vi "WriteAllData.vi"(8 "error in (no error)":errorcluster, 10 "Input":string[](array[string]), 11 "Sensor in":refnum<class "Sensor.lvclass">) -> (0 "error out":errorcluster, 3 "Sensor out":refnum<class "Sensor.lvclass">)   [LabVIEW 2014, in "Sensors.lvlib" / "Sensor.lvclass"]
uses:
  Sensor.lvclass
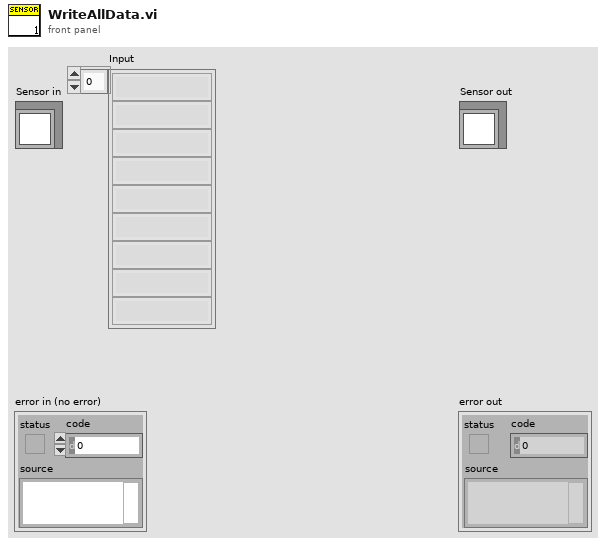
[diagram p1: front panel]
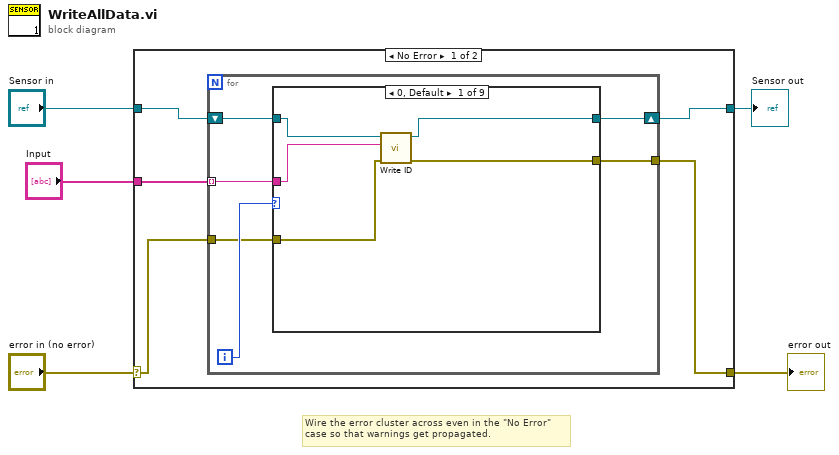
[diagram p0: block diagram]
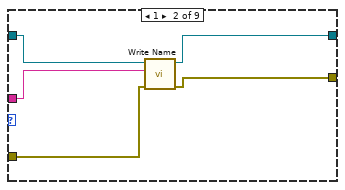
[diagram p2: hidden frame]
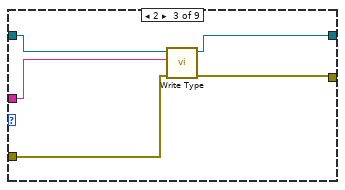
[diagram p3: hidden frame]
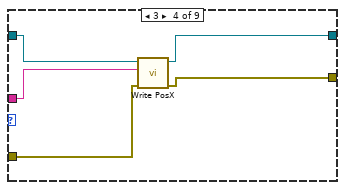
[diagram p4: hidden frame]
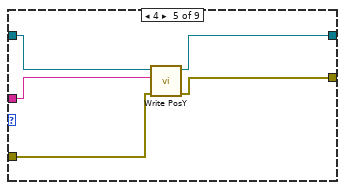
[diagram p5: hidden frame]
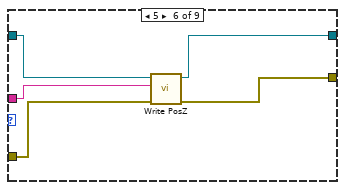
[diagram p6: hidden frame]
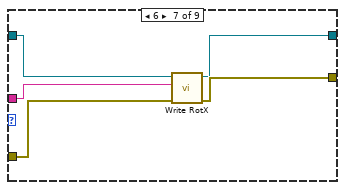
[diagram p7: hidden frame]
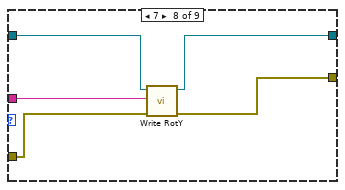
[diagram p8: hidden frame]
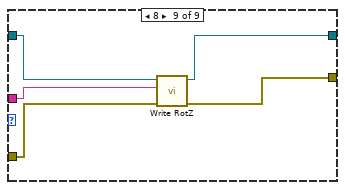
[diagram p9: hidden frame]
diagram:
  # "Wire the error cluster across even in the \"No Error\"\ncase so that warnings get propagated."
  n1 = case shown="No Error" "error in (no error)" {
    selector: "error in (no error)" -> [w7 w63]
    tunnel: [w6 w63] -> w1
    tunnel: [w9 w62] -> w3
    tunnel: "Sensor in" -> [w10 w62]
    tunnel: "Input" -> [w8 _]
    frame No Error {
      n2 = for {
        tunnel: w8 -> [w15] mode=indexing
        tunnel: w7 -> [w12]
        tunnel: [w11] -> w6
        shift-right: [w13] -> w9
        shift-left: w10 -> [w14]
        i -> [w16]
        n3 = case shown="0, Default" w16 {
          tunnel: w15 -> [w19 w24 w29 w35 w40 w45 w50 w53 w59]
          tunnel: w14 -> [w21 w26 w30 w36 w41 w46 w51 w56 w61]
          tunnel: [w20 w25 w31 w33 w38 w43 w47 w55 w60] -> w13
          tunnel: w12 -> [w18 w23 w28 w34 w39 w44 w49 w52 w58]
          tunnel: [w17 w22 w27 w32 w37 w42 w48 w54 w57] -> w11
          frame 0, Default {
            n4 = call "Write ID.vi"("error in (no error)"=w18, "ID"=w19, "Sensor in"=w21) -> ("error out"=w17:errorcluster, "Sensor out"=w20:refnum<class "Sensor.lvclass">)  [unwired: 7 in]
          }
          frame 1 {
            n5 = call "Write Name.vi"("error in (no error)"=w23, "Name"=w24, "Sensor in"=w26) -> ("error out"=w22:errorcluster, "Sensor out"=w25:refnum<class "Sensor.lvclass">)  [unwired: 7 in]
          }
          frame 2 {
            n6 = call "Write Type.vi"("error in (no error)"=w28, "Type"=w29, "Sensor in"=w30) -> ("error out"=w27:errorcluster, "Sensor out"=w31:refnum<class "Sensor.lvclass">)  [unwired: 7 in]
          }
          frame 3 {
            n7 = call "Write PosX.vi"("error in (no error)"=w34, "PosX"=w35, "Sensor in"=w36) -> ("error out"=w32:errorcluster, "Sensor out"=w33:refnum<class "Sensor.lvclass">)  [unwired: 7 in]
          }
          frame 4 {
            n8 = call "Write PosY.vi"("error in (no error)"=w39, "PosY"=w40, "Sensor in"=w41) -> ("error out"=w37:errorcluster, "Sensor out"=w38:refnum<class "Sensor.lvclass">)  [unwired: 7 in]
          }
          frame 5 {
            n9 = call "Write PosZ.vi"("error in (no error)"=w44, "PosZ"=w45, "Sensor in"=w46) -> ("error out"=w42:errorcluster, "Sensor out"=w43:refnum<class "Sensor.lvclass">)  [unwired: 7 in]
          }
          frame 6 {
            n10 = call "Write RotX.vi"("error in (no error)"=w49, "RotX"=w50, "Sensor in"=w51) -> ("error out"=w48:errorcluster, "Sensor out"=w47:refnum<class "Sensor.lvclass">)  [unwired: 7 in]
          }
          frame 7 {
            n11 = call "Write RotY.vi"("error in (no error)"=w52, "RotY"=w53, "Sensor in"=w56) -> ("error out"=w54:errorcluster, "Sensor out"=w55:refnum<class "Sensor.lvclass">)  [unwired: 7 in]
          }
          frame 8 {
            n12 = call "Write RotZ.vi"("error in (no error)"=w58, "RotZ"=w59, "Sensor in"=w61) -> ("error out"=w57:errorcluster, "Sensor out"=w60:refnum<class "Sensor.lvclass">)  [unwired: 7 in]
          }
        }
      }
    }
    frame Error {
    }
  }
  "error out" <- w1
  "Sensor out" <- w3
